vi "Frame Single.vi"() -> ()   [LabVIEW 2021]
uses:
  <userlib>/SciSDK/SciSDK_Labview.lvlib
panel:
  out "Frame Buffer Out":T1
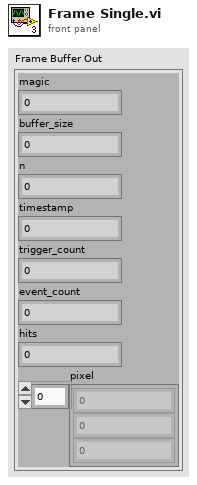
[diagram p1: front panel]
types:
  T1 = cluster{"magic":u32, "buffer_size":u32, "n":u64, "timestamp":u64, "trigger_count":u64, "event_count":u64, "hits":u64, "pixel":u32[]}
  T2 = cluster{"Name":string, "Board Model":string, "Handle":u64}
  T3 = cluster{"Frame Path":string, "Frame Name":string}
  T4 = cluster{"Board Name":string, "Board Model":string, "Handle":u64}
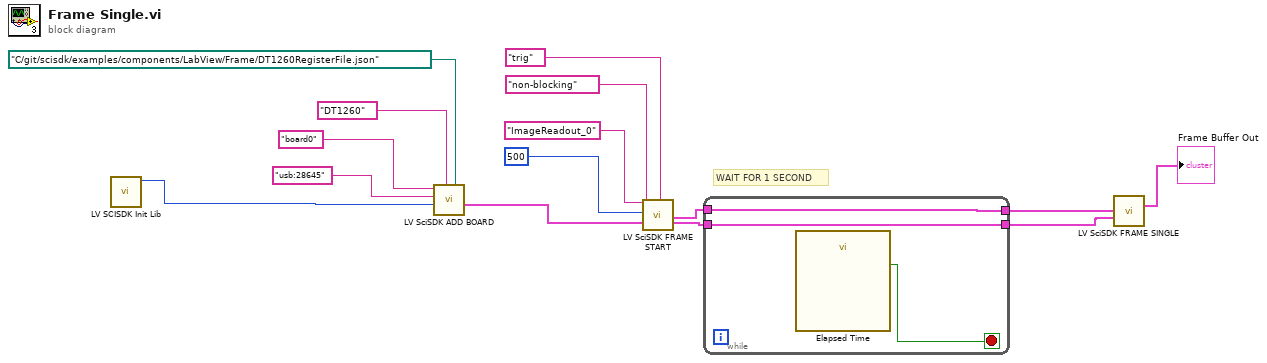
[diagram p0: block diagram]
diagram:
  # "WAIT FOR 1 SECOND"
  n1 = call <userlib>:"LV SCISDK Init Lib.vi"() -> ("function return"=w11:u64)  [unwired: 11 in]
  n2 = call <userlib>:"LV SciSDK ADD BOARD.vi"("JsonFile"=path "C:/git/scisdk/examples/components/LabView/Frame/DT1260RegisterFile.json", "Board Model"="DT1260", "SciSDK Handle"=w11, "DevicePath"="usb:28645", "Name"="board0") -> ("Board Handle Out"=w9:T2)  [unwired: 4 in, 2 out]
  n3 = call <userlib>:"LV SciSDK FRAME START.vi"("Frame Name"="ImageReadout_0", "Acq Mode"="non-blocking", "Timeout"=500, "Board Handle In"=w9, "Trigger Mode"="trig") -> ("Frame Handle Out"=w5:T3, "Board Handle Out"=w4:T4)  [unwired: 12 in, 1 out]
  n4 = while {
    tunnel: w5 -> [w17]
    tunnel: w4 -> [w16]
    tunnel: [w17] -> w2
    tunnel: [w16] -> w3
    stop <- w18 stop-if-true
    n5 = call "Elapsed Time"() -> ("Time has Elapsed"=w18:bool)  [unwired: 12 in, 7 out]
  }
  n6 = call <userlib>:"LV SciSDK FRAME SINGLE.vi"("Frame Handle In"=w2, "Board Handle In"=w3) -> ("Frame Buffer Out"=→"Frame Buffer Out":T1)  [unwired: 9 in, 4 out]
